vi "Load Config.vi"(6 "Constants":refnum<class "Sequence Constants.lvclass">, 8 "error in (no error)":refnum<class "MultiErrors.lvclass">, 10 "Config Element":refnum<class "Config Element.lvclass">, 11 "HTTP Command Config in":refnum<class "HTTP Command Config.lvclass">) -> (0 "error out":refnum<class "MultiErrors.lvclass">, 3 "HTTP Command Config out":refnum<class "HTTP Command Config.lvclass">)   [LabVIEW 2023, in "VolatusSeqConfig.lvlib" / "HTTP Command Config.lvclass"]
uses:
  HTTP Command Config.lvclass
  VolatusErrorUtilities/MultiErrors/MultiErrors.lvclass
  lv-cdm/CDM-Config/Config Element/Config Element.lvclass
  Sequence Constants/Sequence Constants.lvclass
  HTTP Command Config.lvclass/HTTP Command Config.ctl
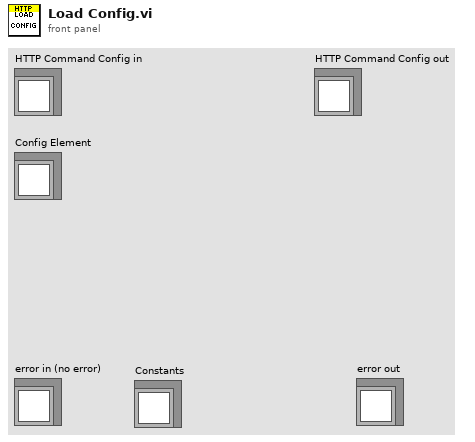
[diagram p1: front panel]
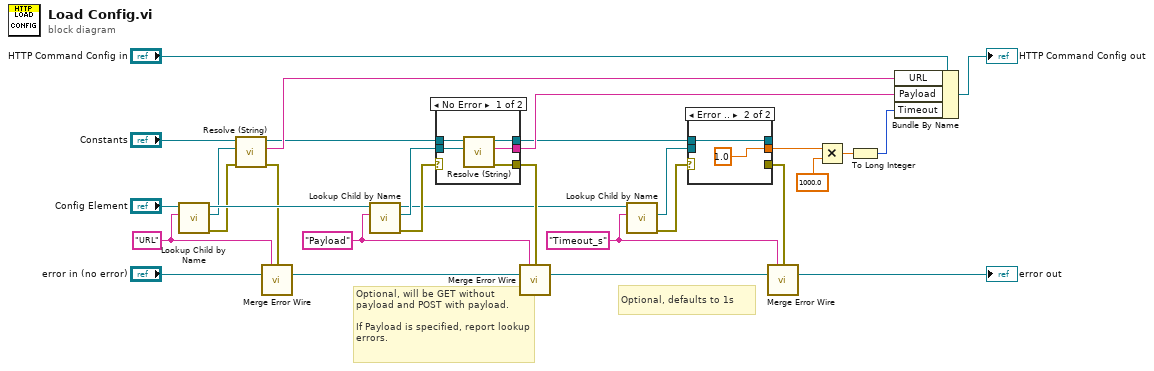
[diagram p0: block diagram]
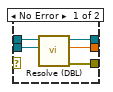
[diagram p2: hidden frame]
diagram:
  w10 = "Timeout_s" ("Name")
  w14 = "Payload" ("Name")
  w13 = "URL" ("Name")
  # "Optional, defaults to 1s"
  # "Optional, will be GET without payload and POST with payload.\n\nIf Payload is specified, report lookup errors."
  n1 = call "Lookup Child by Name.vi"("Name"=w13, "Config Element in"="Config Element") -> ("error out"=w22:errorcluster, "Child"=w23:refnum<class "Config Element.lvclass">, "Config Element out"=w25:refnum<class "Config Element.lvclass">)  [unwired: 6 in, 1 out]
  n2 = call "Resolve (String).vi"("error in (no error)"=w22, "Element"=w23, "Sequence Constants in"="Constants") -> ("error out"=w21:errorcluster, "String Value"=w20:string, "Sequence Constants out"=w19:refnum<class "Sequence Constants.lvclass">)  [unwired: 6 in]
  n3 = call "Merge Error Wire.vi"("Local Context (None)"=w13, "error in (no error)"=w21, "MultiErrors in"="error in (no error)") -> ("MultiErrors out"=w28:refnum<class "MultiErrors.lvclass">)  [unwired: 12 in]
  n4 = call "Lookup Child by Name.vi"("Name"=w14, "Config Element in"=w25) -> ("error out"=w18:errorcluster, "Child"=w17:refnum<class "Config Element.lvclass">, "Config Element out"=w12:refnum<class "Config Element.lvclass">)  [unwired: 6 in, 1 out]
  n5 = case shown="No Error" w18 {
    tunnel: w19 -> [w35 w36]
    tunnel: w17 -> [w34 _]
    tunnel: [w33 _] -> w16
    tunnel: [w32 _] -> w15
    tunnel: [w31 w36] -> w9
    frame No Error {
      n6 = call "Resolve (String).vi"("Element"=w34, "Sequence Constants in"=w35) -> ("error out"=w32:errorcluster, "String Value"=w33:string, "Sequence Constants out"=w31:refnum<class "Sequence Constants.lvclass">)  [unwired: 7 in]
    }
    frame Error {
    }
  }
  n7 = call "Merge Error Wire.vi"("Local Context (None)"=w14, "error in (no error)"=w15, "MultiErrors in"=w28) -> ("MultiErrors out"=w11:refnum<class "MultiErrors.lvclass">)  [unwired: 12 in]
  n8 = call "Lookup Child by Name.vi"("Name"=w10, "Config Element in"=w12) -> ("error out"=w7:errorcluster, "Child"=w8:refnum<class "Config Element.lvclass">)  [unwired: 6 in, 2 out]
  n9 = case shown="Error .." w7 {
    tunnel: w9 -> [w41 w43]
    tunnel: [w37 w43] -> _
    tunnel: w8 -> [w40 _]
    tunnel: [w39 1.0 ("DBL Value")] -> w6
    tunnel: [w38 _] -> w4
    frame No Error {
      n10 = call "Resolve (DBL).vi"("Element"=w40, "Sequence Constants in"=w41) -> ("error out"=w38:errorcluster, "DBL Value"=w39:dbl, "Sequence Constants out"=w37:refnum<class "Sequence Constants.lvclass">)  [unwired: 7 in]
    }
    frame Error {
    }
  }
  n11 = call "Merge Error Wire.vi"("Local Context (None)"=w10, "error in (no error)"=w4, "MultiErrors in"=w11) -> ("MultiErrors out"=→"error out":refnum<class "MultiErrors.lvclass">)  [unwired: 12 in]
  n12 = Multiply(x=w6, y=1000.0) -> (x*y=w2:dbl)
  n13 = To Long Integer(number=w2) -> (32bit integer=w1:i32)
  n14 = Bundle By Name(cluster="HTTP Command Config in", "URL"=w20, "Payload"=w16, "Timeout"=w1) -> (→"HTTP Command Config out":refnum<class "HTTP Command Config.lvclass">)
